vi "Datalogger.vi"() -> ()   [LabVIEW 2025]
uses:
  <vilib>/numeric/Random Number (Range) DBL.vi
  <vilib>/Utility/file.llb/Write Delimited Spreadsheet (DBL).vi
panel:
  out "new file path (Not A Path if cancelled)":path
  in  "file path (dialog if empty)":path=path "C:/Users/vinny/Documents/LabVIEW Data/Test Log Data/Datalog File "
  out "concatenated string":string
  out "appended path":path
  out "Array":dbl[][](array[numeric])
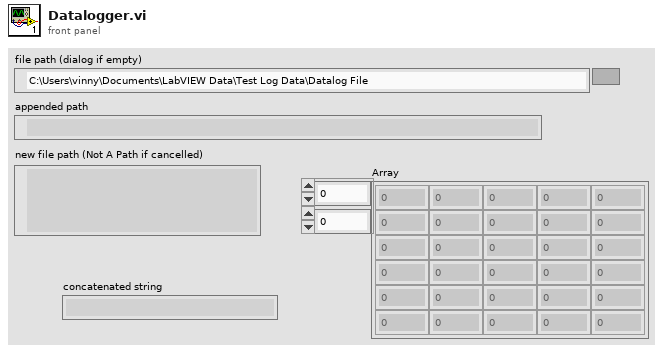
[diagram p1: front panel]
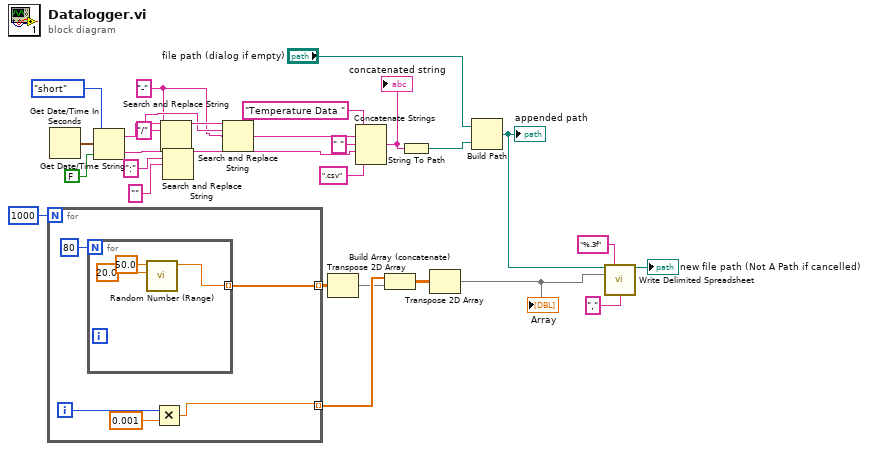
[diagram p0: block diagram]
diagram:
  w6 = "-" ("replace string (\"\")")
  w7 = "/" ("search string")
  n1 = for {
    N: 1000 -> [_]
    tunnel: [w33] -> w23 mode=indexing
    tunnel: [w29] -> w26 mode=indexing
    i -> [w30]
    n2 = for {
      N: 80 -> [_]
      tunnel: [w36] -> w33 mode=indexing
      n3 = call-poly <vilib>:"Random Number (Range).vi"("lower bound (0)"=20.0, "upper bound (100)"=50.0) -> ("number"=w36:dbl)  [unwired: 9 in]
    }
    n4 = Multiply(x=w30, y=0.001) -> (x*y=w29:dbl)
  }
  n5 = Get Date/Time In Seconds() -> (seconds since 1Jan1904=w22:timestamp)
  n6 = Get Date/Time String(date format (0)=enum16{"short", "long", "abbreviated"}."short", seconds (now)=w22, want seconds? (F)=FALSE) -> (date string=w10:string, time string=w14:string)
  n7 = Search and Replace String(input string=w10, search string=w7, replace string=w6) -> (result string=w8:string)  [unwired: 5 in, 3 out]
  n8 = Search and Replace String(input string=w14, search string=":" ("substring (\"\")"), replace string="" ("replace string (\"\")")) -> (result string=w12:string)  [unwired: 5 in, 3 out]
  n9 = Search and Replace String(input string=w8, search string=w7, replace string=w6) -> (result string=w9:string)  [unwired: 5 in, 3 out]
  n10 = Transpose 2D Array(2D array=w23) -> (transposed array=w1:dbl[][])
  n11 = Concatenate Strings("Temperature Data " ("string"), w9, " " ("string"), w12, ".csv" ("string")) -> (w21:string)
  "concatenated string" <- w21
  n12 = Build Array (concatenate)(w26, w1) -> (w27:dbl[][])
  n13 = String To Path(string=w21) -> (path=w18:path)
  n14 = Transpose 2D Array(2D array=w27) -> (transposed array=w2:dbl[][])
  "Array" <- w2
  n15 = Build Path(base path="file path (dialog if empty)", name or relative path=w18) -> (appended path=w5:path)
  "appended path" <- w5
  n16 = call-poly <vilib>:"Write Delimited Spreadsheet.vi"("file path (dialog if empty)"=w5, "format (%.3f)"="%.3f", "2D data"=w2, "delimiter (\\t)"="," ("delimiter (\\t)")) -> ("new file path (Not A Path if cancelled)"=→"new file path (Not A Path if cancelled)":path)  [unwired: 10 in, 1 out]
